vi "Set Oscillator Frequency Sweep Step Frequency.vi"(8 "error in (no error)":errorcluster, 9 "Frequency Sweep Type":T1, 10 "Oscillator Frequency Sweep Step":dbl min=0.0 max=250000.0 step=0.001, 11 "VISA resource name":refnum<visa-resource-name>) -> (0 "error out":errorcluster, 3 "VISA resource name out":refnum<visa-resource-name>)   [LabVIEW 2016, in "SR7270 Drivers.lvlib"]
uses:
  SR7270 Drivers.lvlib
  Typedefs/FSTEP--enum.ctl
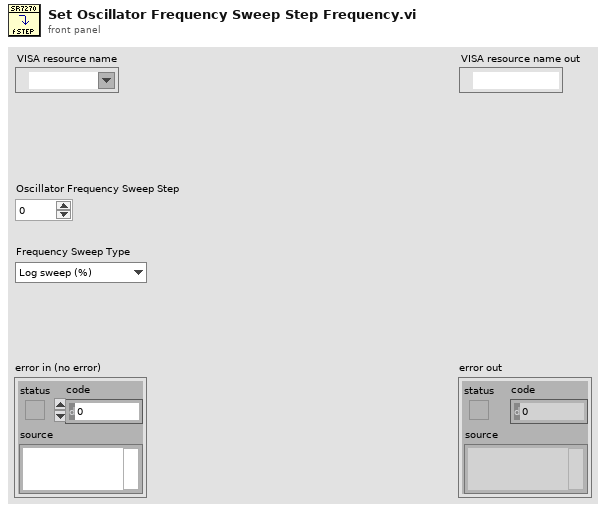
[diagram p1: front panel]
types:
  T1 = typedef "SR7270 Drivers.lvlib/FSTEP--enum.ctl" = enum16{"Log sweep (%)", "Linear sweep (Hz)", "Linear seek sweep (Hz)"}
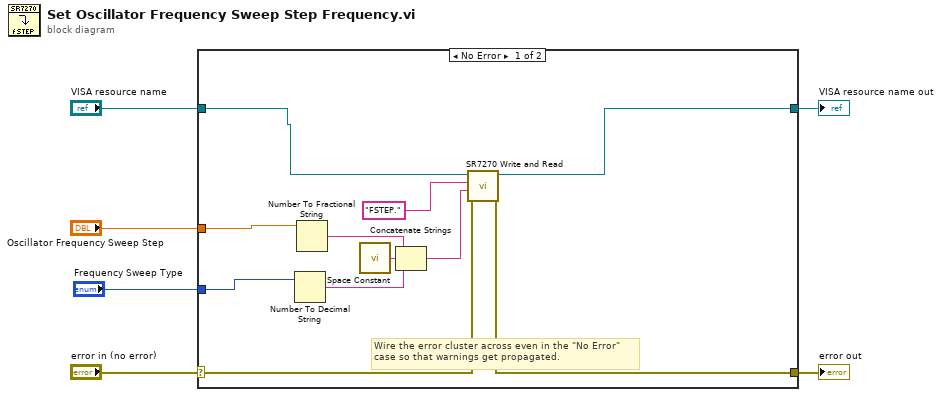
[diagram p0: block diagram]
diagram:
  n1 = case shown="No Error" "error in (no error)" {
    selector: "error in (no error)" -> [w17 w19]
    tunnel: [w16 w19] -> w5
    tunnel: [w8 w18] -> w3
    tunnel: "VISA resource name" -> [w7 w18]
    tunnel: "Oscillator Frequency Sweep Step" -> [w15 _]
    tunnel: "Frequency Sweep Type" -> [w13 _]
    frame No Error {
      # "Wire the error cluster across even in the \"No Error\"\ncase so that warnings get propagated."
      n2 = Number To Decimal String(number=w13) -> (decimal integer string=w10:string)  [unwired: 1 in]
      n3 = Number To Fractional String(number=w15) -> (F-format string=w11:string)  [unwired: 3 in]
      n4 = call <vilib>:"Space Constant.vi"() -> ("String"=w12:string)
      n5 = Concatenate Strings(w11, w12, w10) -> (w9:string)
      n6 = call "SR7270 Write and Read.vi"("error in (no error)"=w17, "Parameter(s)"=w9, "Command Name"="FSTEP.", "VISA resource name"=w7) -> ("error out"=w16:errorcluster, "VISA resource name out"=w8:refnum<visa-resource-name>)  [unwired: 4 in, 2 out]
    }
    frame Error {
    }
  }
  "error out" <- w5
  "VISA resource name out" <- w3
